vi "(SubVI) PSD Calculation_YCC.vi"(4 "sampling frequency (Hz)":i32, 5 "T=NI made PSD\nF=YCC made PSD":bool, 7 "QPD data":dbl[](array[numeric])) -> (2 "Frequency (Hz)\n0,df, 2df,...(n/2-1)Fs":dbl[](array[numeric]), 3 "Power Spectrum (V^2 rms) (V^2/Hz)":dbl[](array[numeric]))   [LabVIEW 2014]
uses:
  <vilib>/Analysis/2dsp.llb/Real FFT.vi
  <vilib>/Analysis/NI_AALPro.lvlib
panel:
  out "Data points":i32
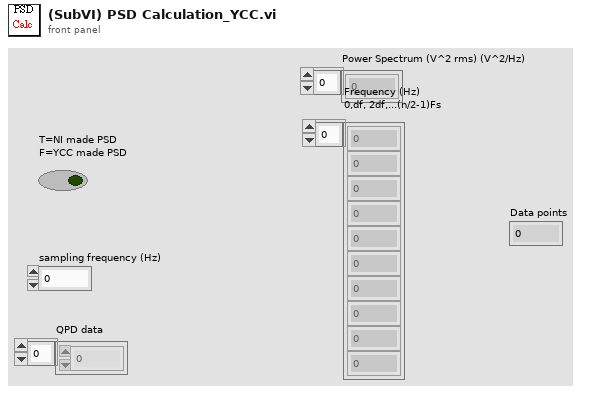
[diagram p1: front panel]
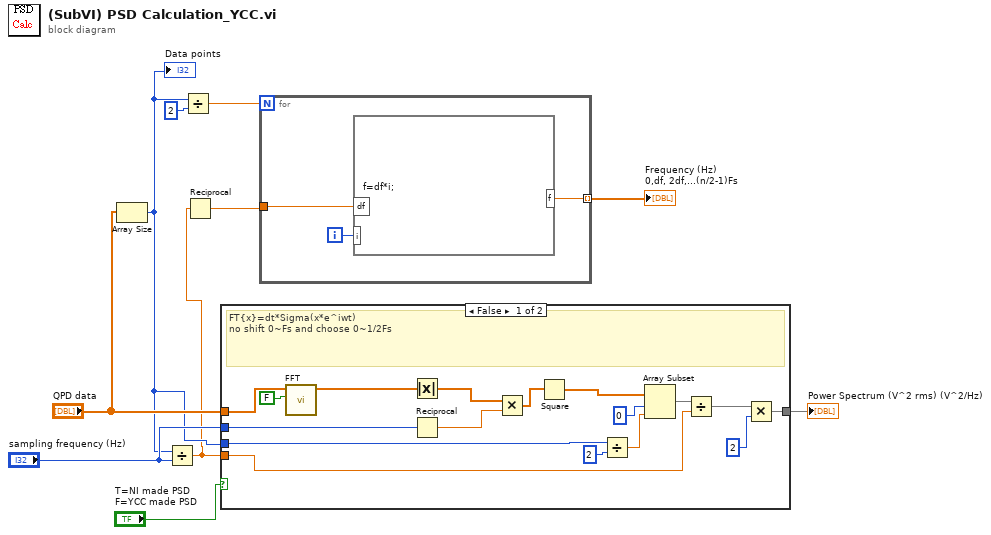
[diagram p0: block diagram]
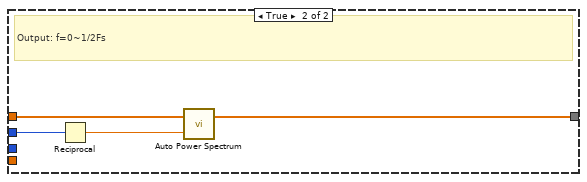
[diagram p2: hidden frame]
diagram:
  n1 = Array Size(array="QPD data") -> (size(s)=w3:i32)
  "Data points" <- w3
  n2 = Divide(x=w3, y="sampling frequency (Hz)") -> (x/y=w2:dbl)
  n3 = Divide(x=w3, y=2) -> (x/y=w6:dbl)
  n4 = Reciprocal(x=w2) -> (1/x=w1:dbl)
  n5 = case shown="False" "T=NI made PSD\nF=YCC made PSD" {
    tunnel: "QPD data" -> [w23 w29]
    tunnel: "sampling frequency (Hz)" -> [w25 w30]
    tunnel: [w16 w28] -> w9
    tunnel: w2 -> [w19 _]
    tunnel: w3 -> [w15 _]
    frame False {
      # "FT{x}=dt*Sigma(x*e^iwt)\nno shift 0~Fs and choose 0~1/2Fs"
      n6 = call-poly <vilib>:"FFT.vi"("shift?"=FALSE, "X"=w23) -> ("FFT {X}"=w26:cdb[])  [unwired: 8 in, 1 out]
      n7 = Absolute Value(x=w26) -> (abs(x)=w14:dbl[])
      n8 = Reciprocal(x=w25) -> (1/x=w13:dbl)
      n9 = Multiply(x=w14, y=w13) -> (x*y=w12:dbl[])
      n10 = Square(x=w12) -> (x^2=w11:dbl[])
      n11 = Divide(x=w15, y=2) -> (x/y=w21:dbl)
      n12 = Array Subset(array=w11, index=0, length=w21) -> (w20:dbl[])
      n13 = Divide(x=w20, y=w19) -> (x/y=w18:dbl[])
      n14 = Multiply(x=w18, y=2) -> (x*y=w16:dbl[])
    }
    frame True {
      # "Output: f=0~1/2Fs"
      n15 = Reciprocal(x=w30) -> (1/x=w31:dbl)
      n16 = call <vilib>:"Auto Power Spectrum.vi"("dt"=w31, "Signal (V)"=w29) -> ("Power Spectrum (V^2 rms)"=w28:dbl[])  [unwired: 1 out]
    }
  }
  "Power Spectrum (V^2 rms) (V^2/Hz)" <- w9
  n17 = for {
    N: w6 -> [_]
    tunnel: w1 -> [w34]
    tunnel: [w32] -> w8 mode=indexing
    i -> [w33]
    n18 = formula code="f=df*i;"("df"=w34, "i"=w33) -> ("f"=w32:dbl)
  }
  "Frequency (Hz)\n0,df, 2df,...(n/2-1)Fs" <- w8
